vi "ExSimpleAsyncNIDisplay.vi"() -> ()   [LabVIEW 2010]
panel:
  out "Image Display":u16[][](graph)
  in  "Trigger Edge":u32(ring)=1 items=["N/A", "Positive (leading) edge", "Negative (falling) edge"]
  in  "Timing Mode":u32(ring)=1 items=["N/A", "Free Run/Timed", "Trigger First (PM only)", "Ext Sync/Strobed ", "Variable Exp (PM only)", "Flash Mode (PM only)"]
  in  "Temperature":dbl format="%.2f"
  in  "Exposure":dbl min=0.0 step=0.001 format="%.3f"
  in  "stop":bool
  in  "Store":bool
  out "error out":errorcluster
  in  "error in (no error)":errorcluster
  # "ExSimipleAsyncNIDisplay:\nThis is a Full Frame Async example, using NI image display. This should work with \nall camera systems. It requires a start for every frame collected. Not all timing modes \nwork for all cameras, also the trigger edge only applies to Princeton Instrument \ncameras. Not all cameras have the ability to set the temperature.\nPressing the stop button stops the example."
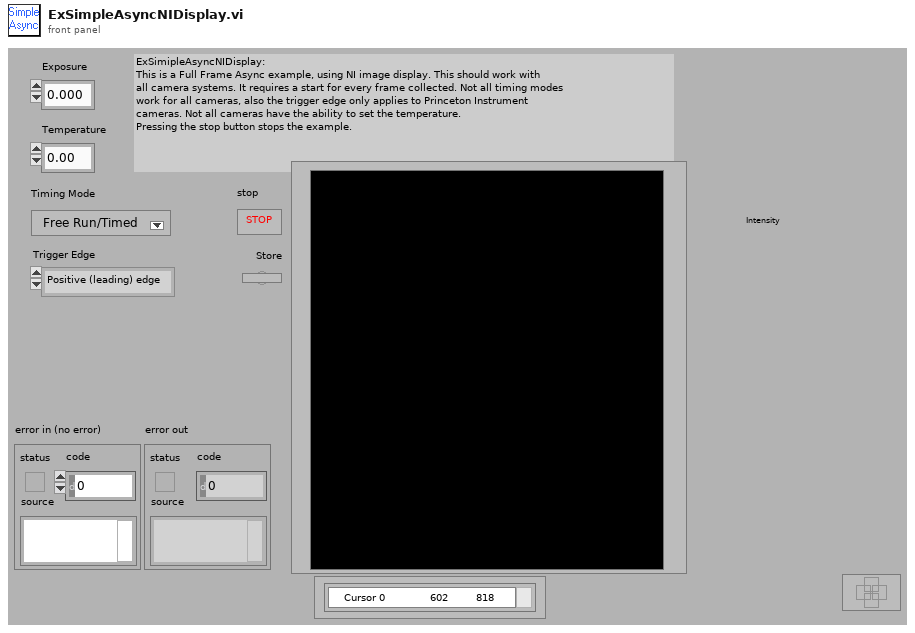
[diagram p1: front panel]
types:
  T1 = cluster{"Acquire mode \n3 is Async":i32, "Exposure":dbl, "Number of Images":i32, "Software Accums":i32}
  T2 = cluster{"Camera Handle":u32, "Pulser Handle":u32, "File Handle":u32, "Display Handle":u32, "Image Handle":u32}
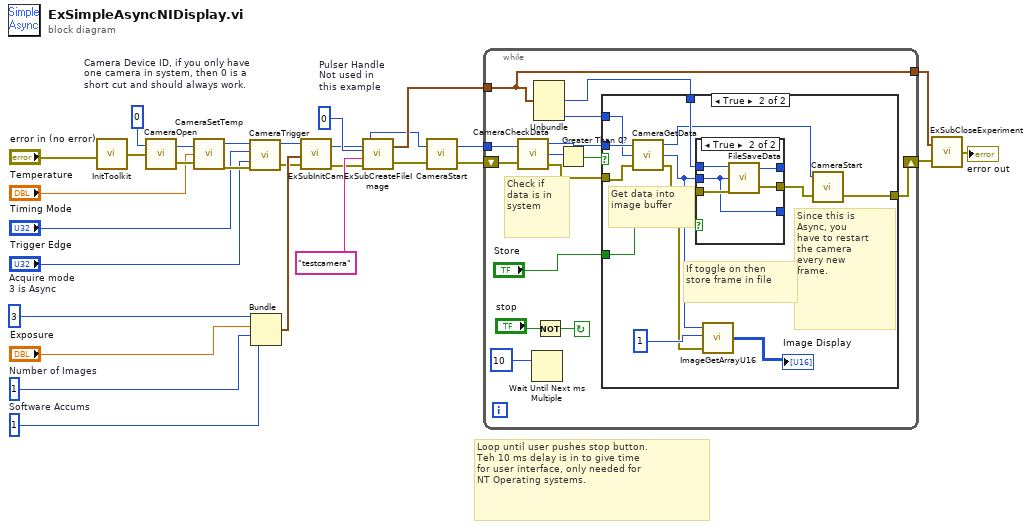
[diagram p0: block diagram]
diagram:
  w14 = 0  # Camera Device ID, if you only have  one camera in system, then 0 is a  short cut and should always work.
  w21 = 0  # Pulser Handle Not used in  this example
  w26 = 1  # Number of Images
  w27 = 3  # Acquire mode  3 is Async
  w25 = 1  # Software Accums
  # "Loop until user pushes stop button.\nTeh 10 ms delay is in to give time \nfor user interface, only needed for \nNT Operating systems."
  n1 = call <userlib>:"InitToolkit.vi"("error in"="error in (no error)") -> ("error out"=w15:errorcluster)
  n2 = call <userlib>:"CameraOpen.vi"("error in"=w15, "Camera Device ID"=w14) -> ("error out"=w12:errorcluster, "Camera Handle"=w13:u32)
  n3 = call <userlib>:"CameraSetTemp.vi"("error in (no error)"=w12, "Temperature"="Temperature", "Camera Handle"=w13) -> ("error out"=w9:errorcluster, "Camera Handle"=w10:u32)
  n4 = call <userlib>:"CameraTrigger.vi"("error in"=w9, "Trigger Edge"="Trigger Edge", "Timing Mode"="Timing Mode", "Camera Handle"=w10) -> ("error out"=w6:errorcluster, "Camera Handle"=w5:u32)
  n5 = Bundle("Acquire mode \n3 is Async"=w27, "Exposure"="Exposure", "Number of Images"=w26, "Software Accums"=w25) -> (w23:T1)  [unwired: 1 in]
  n6 = call "ExSubInitCam.vi"("error in (no error)"=w6, "Camera Information"=w23, "Camera Handle"=w5) -> ("error out"=w22:errorcluster, "Camera Handle"=w18:u32)
  n7 = call "ExSubCreateFileImage.vi"("error in (no error)"=w22, "File and Display Name"="testcamera", "Pulser Handle"=w21, "Camera Handle"=w18) -> ("error out"=w20:errorcluster, "Handles Out"=w19:T2)
  n8 = call <userlib>:"CameraStart.vi"("error in"=w20, "Camera Handle"=w18) -> ("error out"=w3:errorcluster, "Camera Handle"=w4:u32)
  n9 = while {
    tunnel: w19 -> [w29]
    tunnel: w4 -> [w39]
    shift-right: [w33] -> w2
    shift-left: w3 -> [w34]
    tunnel: [w29] -> w1
    stop <- w41 continue-if-true
    # "Check if \ndata is in\nsystem"
    n10 = call <userlib>:"CameraCheckData.vi"("Camera Handle"=w39, "error in"=w34) -> ("Camera Handle"=w36:u32, "Number Of Frames Available"=w38:i32, "error out"=w35:errorcluster)
    n11 = Wait Until Next ms Multiple(millisecond multiple=10) -> ()  [unwired: 1 out]
    n12 = Unbundle(w29) -> ("File Handle"=w32:u32, "Image Handle"=w31:u32)  [unwired: 3 out]
    n13 = Not(x="stop") -> (.not. x?=w41:bool)
    n14 = Greater Than 0?(x=w38) -> (x > 0?=w37:bool)
    n15 = case shown="True" w37 {
      tunnel: w36 -> [_ w55]
      tunnel: w35 -> [w43 w54]
      tunnel: w32 -> [_ w52]
      tunnel: [w43 w50] -> w33
      tunnel: w31 -> [_ w45]
      tunnel: "Store" -> [_ w44]
      frame False {
      }
      frame True {
        # "If toggle on then\nstore frame in file"
        # "Since this is \nAsync, you\nhave to restart \nthe camera\nevery new \nframe."
        # "Get data into\nimage buffer"
        n16 = call <userlib>:"CameraGetData.vi"("error in"=w54, "Data Handle"=w45, "Camera Handle"=w55) -> ("error out"=w46:errorcluster, "Data Handle"=w48:u32, "Camera Handle"=w51:u32)
        n17 = case shown="True" w44 {
          tunnel: [w58 w63] -> _
          tunnel: w46 -> [w57 w62]
          tunnel: w52 -> [w58 w59]
          tunnel: [w57 w61] -> w53
          tunnel: w48 -> [w56 w60]
          tunnel: [w56 w60] -> _
          frame False {
          }
          frame True {
            n18 = call <userlib>:"FileSaveData.vi"("error in"=w62, "Image Handle"=w60, "File Handle"=w59) -> ("error out"=w61:errorcluster, "File Handle"=w63:u32)
          }
        }
        n19 = call <userlib>:"ImageGetArrayU16.vi"("error in"=w46, "Z position"=1, "Image Handle"=w48) -> ("Array uint 16"=→"Image Display":u16[][])  [unwired: 2 out]
        n20 = call <userlib>:"CameraStart.vi"("error in"=w53, "Camera Handle"=w51) -> ("error out"=w50:errorcluster)  [unwired: 1 out]
      }
    }
  }
  n21 = call "ExSubCloseExperiment.vi"("error in (no error)"=w2, "Handles In"=w1) -> ("error out"=→"error out":errorcluster)
